vi "Take Comp Data.vi"(0 "Maximum V_Inject":dbl format="%.4f", 1 "Tolerence":dbl format="%.4f", 2 "Output Terminals(+6 V:0)":u16(ring) items=["+6 V output", "+25 V output", "-25 V output"], 3 "Nominal Frequency":dbl format="%.2f", 4 "Output File":path, 6 "Oscillator Under Test":u16=1 min=1 max=80, 7 "Minimum V_Inject":dbl format="%.4f", 8 "Dmm Readings":i8=1 min=1 max=8, 9 "Frequency Channel":enum16{"Channel 1", "Channel 2", "Channel 3"}(ring), 10 "Gate Time":T1(ring)=enum."1.0 second") -> ()   [LabVIEW 2024]
panel:
  out "Multimeter Address":u8=1 min=1 max=31
  out "PowerSupplyType":i32
  out "Power Supply Address":u8=5
  out "Frequency Counter Address":i16=3 max=31
  out "V_inject":dbl[](array[numeric]) format="%.6f"
  out "Iteration Successful":bool[](array[boolean])
  out "Error":dbl[](array[numeric]) format="%.2f"
  out "Measured Frequency":dbl[](array[numeric]) format="%.6f"
  out "Pullability":dbl[](array[numeric]) format="%.6f"
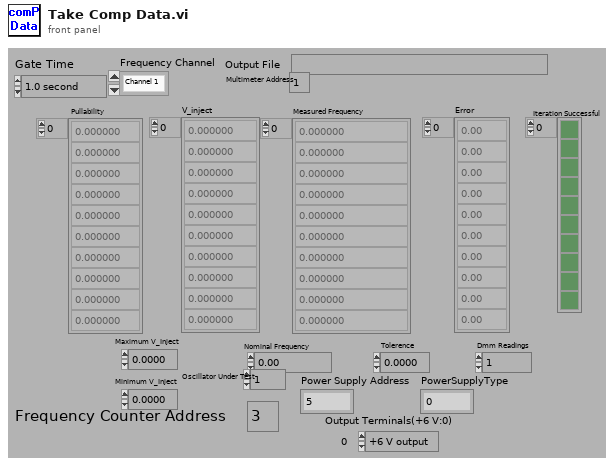
[diagram p1: front panel]
types:
  T1 = enum16{"0.1 second", "1.0 second", "10.0 second"}
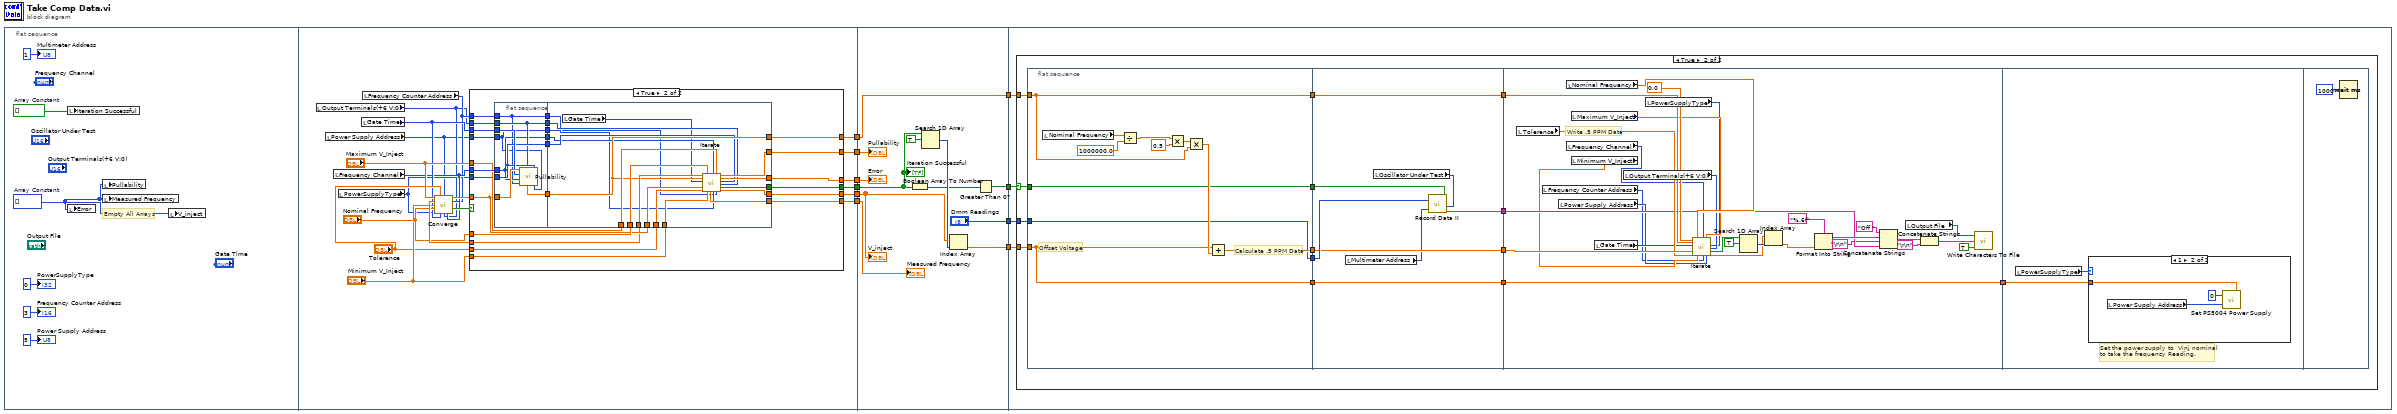
[diagram p0: block diagram]
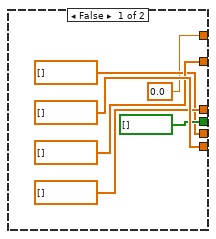
[diagram p2: hidden frame]
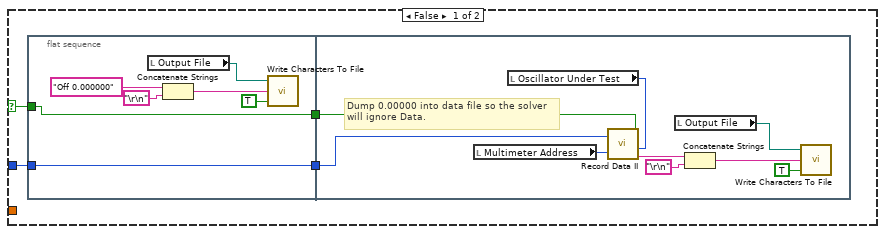
[diagram p3: hidden frame]
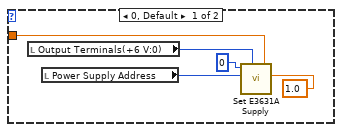
[diagram p4: hidden frame]
diagram:
  n1 = flat-sequence {
    tunnel: [w31] -> w10
    tunnel: [w30] -> w9
    tunnel: [w29] -> w8
    tunnel: [w28] -> w7
    tunnel: [w27] -> w6
    tunnel: [w26] -> w5
    tunnel: w10 -> [w97]
    tunnel: w9 -> [w96]
    tunnel: w8 -> [w95]
    tunnel: w7 -> [w98]
    tunnel: w6 -> [w100]
    tunnel: w5 -> [w103]
    tunnel: [w103] -> w4
    tunnel: [w94] -> w3
    tunnel: [w93] -> w2
    tunnel: ["Dmm Readings"] -> w1
    tunnel: w4 -> [w106]
    tunnel: w3 -> [w105]
    tunnel: w2 -> [w107]
    tunnel: w1 -> [w104]
    frame #0 {
      w15 = bool[] []  # Array Constant
      w16 = i32[] []  # Array Constant
      # "Empty All Arrays"
      n2 = local write "Iteration Successful"(w15) -> ()
      n3 = local write "Error"(w16) -> ()
      n4 = local write "Pullability"(w16) -> ()
      n5 = local write "Measured Frequency"(w16) -> ()
      n6 = local write "V_inject"(w16) -> ()
      "Frequency Counter Address" <- i16 3 ("Frequency Counter Address")
      "Power Supply Address" <- u8 5 ("Power Supply Address")
      "PowerSupplyType" <- 0 ("PowerSupplyType")
      "Multimeter Address" <- u8 1 ("Multimeter Address")
    }
    frame #1 {
      n7 = local read "Output Terminals(+6 V:0)"() -> (w19:u16)
      n8 = local read "Power Supply Address"() -> (w17:u8)
      n9 = local read "Frequency Channel"() -> (w21:enum16{"Channel 1", "Channel 2", "Channel 3"})
      n10 = local read "PowerSupplyType"() -> (w18:i32)
      n11 = local read "Gate Time"() -> (w22:T1)
      n12 = local read "Frequency Counter Address"() -> (w20:i16)
      n13 = call "Converge.vi"("Maximum V_Inject"="Maximum V_Inject", "Tolerence"="Tolerence", "Power Supply Address"=w17, "Frequency Counter Address"=w20, "Minimum V_Inject"="Minimum V_Inject", "Nominal Frequency"="Nominal Frequency", "PowerSupplyType"=w18, "Gate Time"=w22, "Output Terminals(+6 V:0)"=w19, "Frequency Channel"=w21) -> ("V_Inject"=w34:dbl, "Min Error"=w33:dbl, "Converge OK!"=w35:bool)  [unwired: 1 in, 2 out]
      n14 = case shown="True" w35 {
        tunnel: w34 -> [_ w57]
        tunnel: "Tolerence" -> [_ w58]
        tunnel: w33 -> [_ w55]
        tunnel: "Nominal Frequency" -> [_ w59]
        tunnel: [dbl[] [] ("Measured Frequency") w50] -> w31
        tunnel: [dbl[] [] ("Pullability") w51] -> w30
        tunnel: [dbl[] [] ("Error") w52] -> w29
        tunnel: [bool[] [] ("Iteration Successful") w53] -> w28
        tunnel: [dbl[] [] ("V_inject") w54] -> w27
        tunnel: [0.0 ("Pullability") w56] -> w26
        tunnel: "Minimum V_Inject" -> [_ w60]
        tunnel: "Maximum V_Inject" -> [_ w61]
        tunnel: w22 -> [_ w65]
        tunnel: w21 -> [_ w64]
        tunnel: w20 -> [_ w63]
        tunnel: w19 -> [_ w62]
        tunnel: w18 -> [_ w48]
        tunnel: w17 -> [_ w49]
        frame False {
        }
        frame True {
          n15 = flat-sequence {
            tunnel: w57 -> [w73]
            tunnel: w65 -> [w72]
            tunnel: w64 -> [w68]
            tunnel: w63 -> [w67]
            tunnel: w62 -> [w69]
            tunnel: w49 -> [w66]
            tunnel: w48 -> [w70]
            tunnel: [w71] -> w47
            tunnel: [w70] -> w46
            tunnel: [w69] -> w45
            tunnel: [w68] -> w44
            tunnel: [w67] -> w43
            tunnel: [w66] -> w42
            tunnel: w61 -> [w91]
            tunnel: w60 -> [w90]
            tunnel: w59 -> [w89]
            tunnel: w58 -> [w88]
            tunnel: w57 -> [w87]
            tunnel: [w80] -> w56
            tunnel: w55 -> [w86]
            tunnel: [w85] -> w54
            tunnel: [w84] -> w53
            tunnel: [w83] -> w52
            tunnel: [w82] -> w51
            tunnel: [w81] -> w50
            tunnel: w47 -> [w80]
            tunnel: w46 -> [w79]
            tunnel: w45 -> [w78]
            tunnel: w44 -> [w77]
            tunnel: w43 -> [w76]
            tunnel: w42 -> [w75]
            frame #0 {
              n16 = call "Pullability.vi"("Power Supply Address"=w66, "PowerSupplyType"=w70, "Output Terminals(+6 V:0)"=w69, "Frequency Counter Address"=w67, "Frequency Channel"=w68, "Gate Time"=w72, "Ideal V_inj"=w73) -> ("Pullability"=w71:dbl)
            }
            frame #1 {
              n17 = local read "Gate Time"() -> (w74:T1)
              n18 = call "Iterate.vi"("Initial Error"=w86, "Initial Pullability"=w80, "Gate Time"=w74, "V_inject Initial"=w87, "Tolerence"=w88, "Frequency"=w89, "V Low Limit"=w90, "Frequency Channel"=w77, "Frequency Address"=w76, "V High Limit"=w91, "Power Supply Address"=w75, "PowerSupplyType"=w79, "Output Terminals(+6 V:0)"=w78) -> ("Measured Frequency"=w81:dbl[], "Pullability"=w82:dbl[], "Error"=w83:dbl[], "Iteration Successful"=w84:bool[], "V_inject"=w85:dbl[])  [unwired: 2 in]
            }
          }
        }
      }
    }
    frame #2 {
      n19 = Boolean Array To Number(Boolean array=w98) -> (number=w101:u32)
      n20 = Search 1D Array(1D array=w98, element=TRUE) -> (index of element=w102:i32)  [unwired: 1 in]
      n21 = Index Array(array=w100, index=w102) -> (element=w94:dbl)
      n22 = Greater Than 0?(x=w101) -> (x > 0?=w93:bool)
      "V_inject" <- w100
      "Iteration Successful" <- w98
      "Error" <- w95
      "Pullability" <- w96
      "Measured Frequency" <- w97
    }
    frame #3 {
      n23 = case shown="True" w107 {
        selector: w107 -> [w111 w139]
        tunnel: w106 -> [_ w141]
        tunnel: w105 -> [_ w140]
        tunnel: w104 -> [w110 w138]
        frame False {
          n24 = flat-sequence {
            tunnel: w111 -> [w118]
            tunnel: [w118] -> w109
            tunnel: w110 -> [w117]
            tunnel: [w117] -> w108
            tunnel: w109 -> [w127]
            tunnel: w108 -> [w126]
            frame #0 {
              n25 = local read "Output File"() -> (w112:path)
              n26 = Concatenate Strings("Off 0.000000" ("String"), "\r\n") -> (w115:string)
              n27 = call "Write Characters To File.vi"("append to file? (new file:F)"=TRUE, "character string"=w115, "file path (dialog if empty)"=w112) -> ()  [unwired: 2 in, 1 out]
            }
            frame #1 {
              # "Dump 0.00000 into data file so the solver\nwill ignore Data."
              n28 = local read "Multimeter Address"() -> (w119:u8)
              n29 = local read "Oscillator Under Test"() -> (w120:u16)
              n30 = call "Record Data II.vi"("Oscillator Under Test"=w120, "Iteration Successful"=w127, "Multimeter Address"=w119, "Number of Dmm Readings"=w126) -> ("Dmm Readings"=w122:string)  [unwired: 2 in]
              n31 = local read "Output File"() -> (w121:path)
              n32 = Concatenate Strings(w122, "\r\n") -> (w124:string)
              n33 = call "Write Characters To File.vi"("append to file? (new file:F)"=TRUE, "character string"=w124, "file path (dialog if empty)"=w121) -> ()  [unwired: 2 in, 1 out]
            }
          }
        }
        frame True {
          n34 = flat-sequence {
            tunnel: w141 -> [w147]
            tunnel: [w147] -> w137
            tunnel: w140 -> [w144]
            tunnel: w139 -> [w143]
            tunnel: [w143] -> w136
            tunnel: w138 -> [w142]
            tunnel: [w142] -> w135
            tunnel: [w146] -> w134
            tunnel: [w144] -> w133
            tunnel: w137 -> [w157]
            tunnel: [w157] -> w132
            tunnel: w136 -> [w160]
            tunnel: w135 -> [w159]
            tunnel: w134 -> [w156]
            tunnel: [w156] -> w131
            tunnel: [w158] -> w130
            tunnel: w133 -> [w155]
            tunnel: [w155] -> w129
            tunnel: w132 -> [w183]
            tunnel: w131 -> [w186]
            tunnel: w130 -> [w181]
            tunnel: w129 -> [w177]
            tunnel: [w177] -> w128
            tunnel: w128 -> [w190]
            frame #0 {
              # "Offset Voltage"
              # "Calculate .5 PPM Data"
              n35 = local read "Nominal Frequency"() -> (w151:dbl)
              n36 = Divide(x=w151, y=1000000.0) -> (x/y=w150:dbl)
              n37 = Multiply(x=w150, y=0.5) -> (x*y=w148:dbl)
              n38 = Multiply(x=w148, y=w147) -> (x*y=w145:dbl)
              n39 = Add(x=w144, y=w145) -> (x+y=w146:dbl)
            }
            frame #1 {
              n40 = local read "Multimeter Address"() -> (w153:u8)
              n41 = local read "Oscillator Under Test"() -> (w154:u16)
              n42 = call "Record Data II.vi"("Oscillator Under Test"=w154, "Iteration Successful"=w160, "Multimeter Address"=w153, "Number of Dmm Readings"=w159) -> ("Dmm Readings"=w158:string)  [unwired: 2 in]
            }
            frame #2 {
              # "Write .5 PPM Data"
              n43 = local read "Tolerence"() -> (w184:dbl)
              n44 = local read "Frequency Counter Address"() -> (w162:i16)
              n45 = local read "Power Supply Address"() -> (w164:u8)
              n46 = local read "Nominal Frequency"() -> (w185:dbl)
              n47 = local read "Frequency Channel"() -> (w161:enum16{"Channel 1", "Channel 2", "Channel 3"})
              n48 = local read "Maximum V_Inject"() -> (w179:dbl)
              n49 = local read "Minimum V_Inject"() -> (w178:dbl)
              n50 = local read "Gate Time"() -> (w166:T1)
              n51 = local read "Output Terminals(+6 V:0)"() -> (w165:u16)
              n52 = local read "PowerSupplyType"() -> (w163:i32)
              n53 = call "Iterate.vi"("Initial Error"=0.0, "Initial Pullability"=w183, "Gate Time"=w166, "V_inject Initial"=w186, "Tolerence"=w184, "Frequency"=w185, "V Low Limit"=w178, "Frequency Channel"=w161, "Frequency Address"=w162, "V High Limit"=w179, "Power Supply Address"=w164, "PowerSupplyType"=w163, "Output Terminals(+6 V:0)"=w165) -> ("Iteration Successful"=w170:bool[], "V_inject"=w168:dbl[])  [unwired: 2 in, 3 out]
              n54 = Search 1D Array(1D array=w170, element=TRUE) -> (index of element=w169:i32)  [unwired: 1 in]
              n55 = Index Array(array=w168, index=w169) -> (element=w167:dbl)
              n56 = Format Into String(format string="%.6f" ("Format String"), w167) -> (resulting string=w187:string)  [unwired: 2 in, 1 out]
              n57 = Concatenate Strings("Off " ("Substring"), w187, "\r\n", w181) -> (w173:string)
              n58 = local read "Output File"() -> (w172:path)
              n59 = Concatenate Strings(w173, "\r\n") -> (w176:string)
              n60 = call "Write Characters To File.vi"("append to file? (new file:F)"=TRUE, "character string"=w176, "file path (dialog if empty)"=w172) -> ()  [unwired: 2 in, 1 out]
            }
            frame #3 {
              # "Set the power supply to  Vinj nominal\nto take the frequency Reading."
              n61 = local read "PowerSupplyType"() -> (w191:i32)
              n62 = case shown="1" w191 {
                tunnel: w190 -> [w196 w198]
                frame 0, Default {
                  n63 = local read "Output Terminals(+6 V:0)"() -> (w193:u16)
                  n64 = local read "Power Supply Address"() -> (w194:u8)
                  n65 = call "Set E3631A Supply.vi"("Current Limit"=1.0, "Voltage Limit"=w196, "Output Terminals(+6 V:0)"=w193, "Address"=w194, "GPIB#"=u8 0) -> ()  [unwired: 3 in, 1 out]
                }
                frame 1 {
                  n66 = local read "Power Supply Address"() -> (w197:u8)
                  n67 = call "Set PS5004 Power Supply.vi"("Voltage"=w198, "Address"=w197, "System#"=0) -> ()
                }
              }
            }
            frame #4 {
              n68 = Wait (ms)(milliseconds to wait=u32 1000) -> ()  [unwired: 1 out]
            }
          }
        }
      }
    }
  }
